vi "get screen size.vi"(4 "screen":i32) -> (0 "wind size (width/height)":T1, 1 "height":i16, 2 "width":i16)   [LabVIEW 2011]
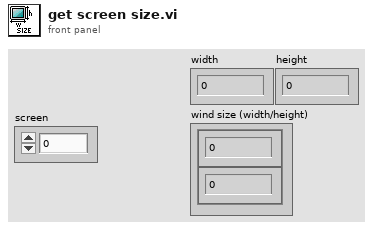
[diagram p1: front panel]
types:
  T1 = cluster{"Numeric Control":i16, "Numeric Control":i16}
  T2 = typedef "LVAllMonitorsDisplayTypeDef.ctl" = cluster{"Bounds":cluster{"Left":i16, "Top":i16, "Right":i16, "Bottom":i16}, "Depth":i16}[]
  T3 = cluster{"Bounds":cluster{"Left":i16, "Top":i16, "Right":i16, "Bottom":i16}, "Depth":i16}
  T4 = cluster{"Left":i16, "Top":i16, "Right":i16, "Bottom":i16}
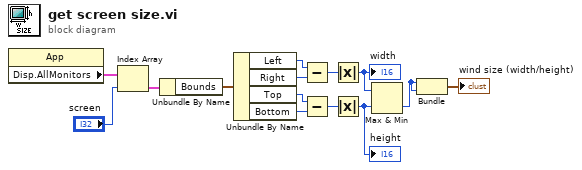
[diagram p0: block diagram]
diagram:
  n1 = property class="App"() -> ("Disp.AllMonitors"=w14:T2)  [unwired: 2 in, 2 out]
  n2 = Index Array(array=w14, index="screen") -> (element=w6:T3)
  n3 = Unbundle By Name(w6) -> ("Bounds"=w13:T4)
  n4 = Unbundle By Name(w13) -> ("Left"=w12:i16, "Right"=w9:i16, "Top"=w8:i16, "Bottom"=w7:i16)
  n5 = Subtract(x=w12, y=w9) -> (x-y=w11:i16)
  n6 = Subtract(x=w8, y=w7) -> (x-y=w10:i16)
  n7 = Absolute Value(x=w11) -> (abs(x)=w3:i16)
  "width" <- w3
  n8 = Absolute Value(x=w10) -> (abs(x)=w2:i16)
  "height" <- w2
  n9 = Max & Min(x=w3, y=w2) -> (min(x,y)=w1:i16)  [unwired: 1 out]
  n10 = Bundle(w1, w1) -> (→"wind size (width/height)":cluster{i16, i16})  [unwired: 1 in]
